vi "Generate intial guess.vi"(2 "数组":dbl[][](array[numeric])) -> (14 "peak":dbl, 15 "xc":dbl, 16 "yc":dbl, 17 "sigx":i32, 18 "sigy":i32)   [LabVIEW 2015]
panel:
  out "sum":dbl
  out "数组 3":ext[](array[numeric])
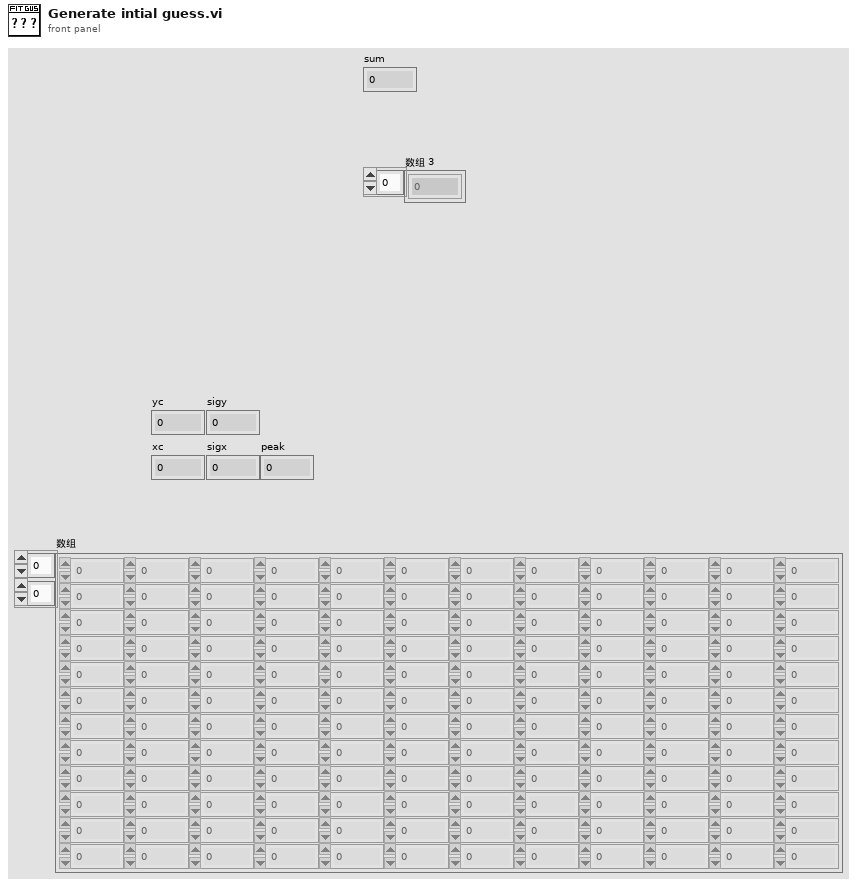
[diagram p1: front panel]
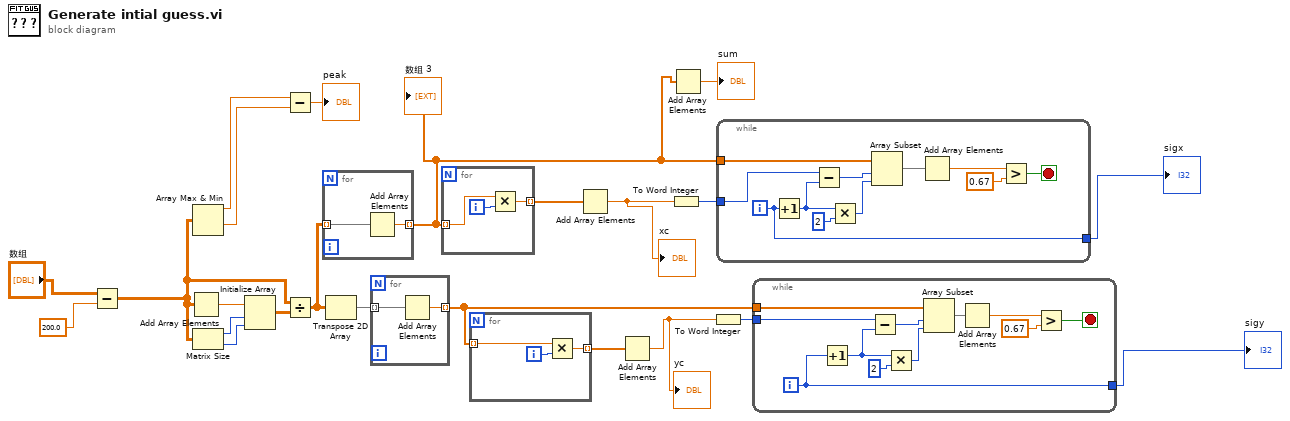
[diagram p0: block diagram]
diagram:
  n1 = Subtract(x="数组", y=200.0) -> (x-y=w3:dbl[][])
  n2 = Add Array Elements(numeric array=w3) -> (sum=w21:dbl)
  n3 = Array Max & Min(array=w3) -> (max value=w12:dbl, min value=w11:dbl)  [unwired: 2 out]
  n4 = Matrix Size(0:w3) -> (1:w23:i32, 2:w22:i32)
  n5 = Initialize Array(w21, w23, w22) -> (w20:dbl[][])
  n6 = Subtract(x=w12, y=w11) -> (x-y=→"peak":dbl)
  n7 = Divide(x=w3, y=w20) -> (x/y=w19:dbl[][])
  n8 = for {
    tunnel: w19 -> [w25] mode=indexing
    tunnel: [w24] -> w2 mode=indexing
    n9 = Add Array Elements(numeric array=w25) -> (sum=w24:dbl)
  }
  "数组 3" <- w2
  n10 = Transpose 2D Array(2D array=w19) -> (transposed array=w18:dbl[][])
  n11 = for {
    tunnel: w18 -> [w27] mode=indexing
    tunnel: [w26] -> w14 mode=indexing
    n12 = Add Array Elements(numeric array=w27) -> (sum=w26:dbl)
  }
  n13 = for {
    tunnel: w2 -> [w29] mode=indexing
    tunnel: [w28] -> w16 mode=indexing
    i -> [w30]
    n14 = Multiply(x=w29, y=w30) -> (x*y=w28:dbl)
  }
  n15 = for {
    tunnel: w14 -> [w32] mode=indexing
    tunnel: [w31] -> w17 mode=indexing
    i -> [w33]
    n16 = Multiply(x=w32, y=w33) -> (x*y=w31:dbl)
  }
  n17 = Add Array Elements(numeric array=w16) -> (sum=w9:dbl)
  "xc" <- w9
  n18 = Add Array Elements(numeric array=w17) -> (sum=w8:dbl)
  "yc" <- w8
  n19 = To Word Integer(number=w9) -> (16bit integer=w13:i16)
  n20 = Add Array Elements(numeric array=w2) -> (sum=→"sum":dbl)
  n21 = To Word Integer(number=w8) -> (16bit integer=w15:i16)
  n22 = while {
    tunnel: w13 -> [w44]
    tunnel: w2 -> [w39]
    tunnel: [w34] -> w7
    i -> [w34]
    stop <- w35 stop-if-true
    n23 = Increment(x=w34) -> (x+1=w42:i32)
    n24 = Subtract(x=w44, y=w42) -> (x-y=w43:i32)
    n25 = Multiply(x=w42, y=2) -> (x*y=w40:i32)
    n26 = Array Subset(array=w39, index=w43, length=w40) -> (w38:dbl[])
    n27 = Add Array Elements(numeric array=w38) -> (sum=w37:dbl)
    n28 = Greater?(x=w37, y=0.67) -> (0:w35:bool)
  }
  "sigx" <- w7
  n29 = while {
    tunnel: w15 -> [w55]
    tunnel: w14 -> [w50]
    tunnel: [w45] -> w6
    i -> [w45]
    stop <- w46 stop-if-true
    n30 = Increment(x=w45) -> (x+1=w53:i32)
    n31 = Subtract(x=w55, y=w53) -> (x-y=w54:i32)
    n32 = Multiply(x=w53, y=2) -> (x*y=w51:i32)
    n33 = Array Subset(array=w50, index=w54, length=w51) -> (w49:dbl[])
    n34 = Add Array Elements(numeric array=w49) -> (sum=w48:dbl)
    n35 = Greater?(x=w48, y=0.67) -> (0:w46:bool)
  }
  "sigy" <- w6
